vi "chr63204A_Error_conversion.vi"(8 "error in (no error)":errorcluster, 11 "VISA resource name":refnum<visa-resource-name>) -> (0 "error out":errorcluster, 3 "VISA resource name out":refnum<visa-resource-name>)   [LabVIEW 2020]
doc: "This VI converts chr63204A machine errors to LabView errors"
panel:
  out "PROT?":bool[](array[boolean])
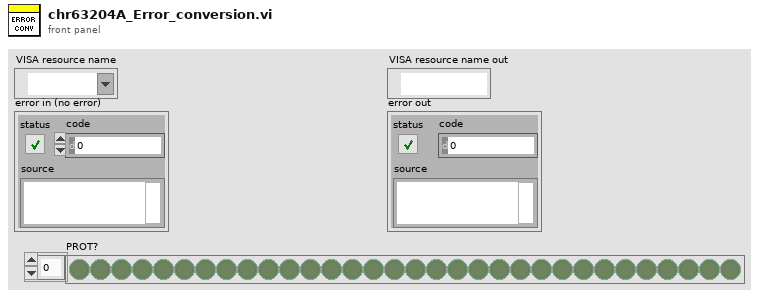
[diagram p1: front panel]
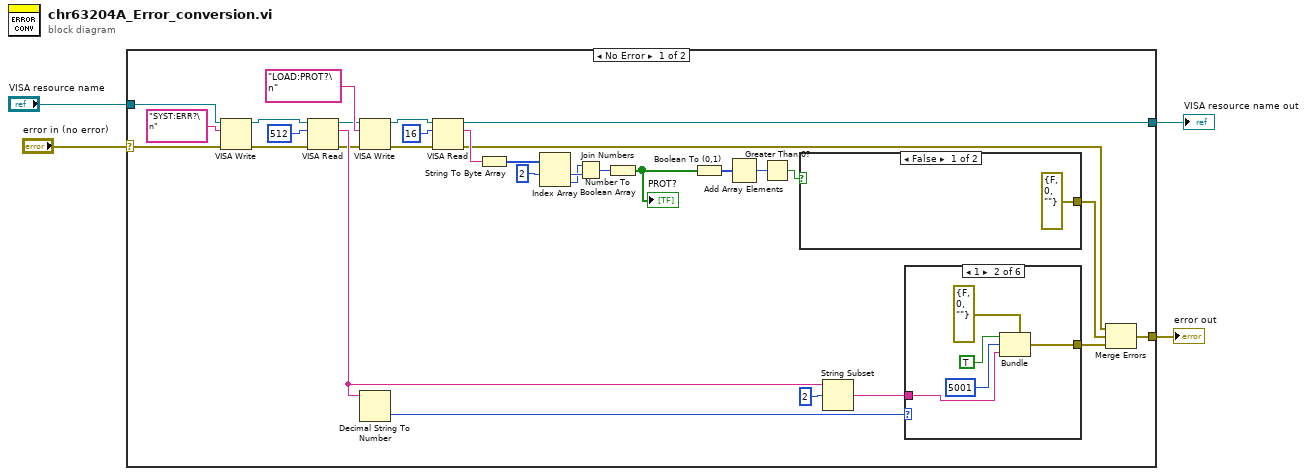
[diagram p0: block diagram]
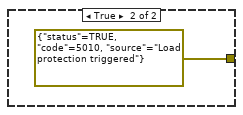
[diagram p2: hidden frame]
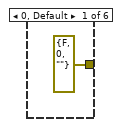
[diagram p3: hidden frame]
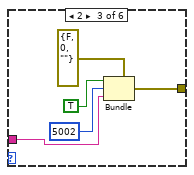
[diagram p4: hidden frame]
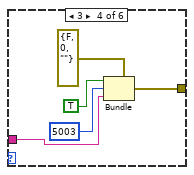
[diagram p5: hidden frame]
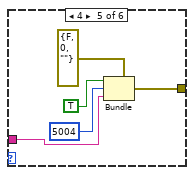
[diagram p6: hidden frame]
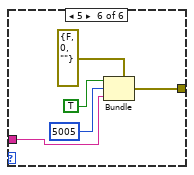
[diagram p7: hidden frame]
diagram:
  n1 = case shown="No Error" "error in (no error)" {
    selector: "error in (no error)" -> [w26 w64]
    tunnel: "VISA resource name" -> [w30 w65]
    tunnel: [w24 w64] -> w1
    tunnel: [w8 w65] -> w2
    frame No Error {
      n2 = VISA Write(VISA resource name=w30, write buffer="SYST:ERR?\n" ("Write Buffer"), error in (no error)=w26) -> (VISA resource name out=w29:refnum<visa-resource-name>, error out=w28:errorcluster)  [unwired: 1 out]
      n3 = VISA Read(VISA resource name=w29, byte count=u32 512, error in (no error)=w28) -> (VISA resource name out=w9:refnum<visa-resource-name>, read buffer=w27:string, error out=w10:errorcluster)  [unwired: 1 out]
      n4 = VISA Write(VISA resource name=w9, write buffer="LOAD:PROT?\n", error in (no error)=w10) -> (VISA resource name out=w21:refnum<visa-resource-name>, error out=w20:errorcluster)  [unwired: 1 out]
      n5 = Decimal String To Number(string=w27) -> (number=w35:i32)  [unwired: 2 in, 1 out]
      n6 = VISA Read(VISA resource name=w21, byte count=u32 16, error in (no error)=w20) -> (VISA resource name out=w8:refnum<visa-resource-name>, read buffer=w18:string, error out=w5:errorcluster)  [unwired: 1 out]
      n7 = String To Byte Array(string=w18) -> (unsigned byte array=w23:u8[])
      n8 = Index Array(array=w23, index #1=2 ("y")) -> (element #1=w22:u8, element #2=w16:u8)  [unwired: 1 in]
      n9 = Join Numbers(hi=w16, lo=w22) -> ((hi.lo)=w15:u16)
      n10 = Number To Boolean Array(number=w15) -> (Boolean array=w14:bool[])
      "PROT?" <- w14
      n11 = Boolean To (0,1)(Boolean=w14) -> (0, 1=w13:i16[])
      n12 = Add Array Elements(numeric array=w13) -> (sum=w12:i16)
      n13 = Greater Than 0?(x=w12) -> (x > 0?=w7:bool)
      n14 = case shown="False" w7 {
        tunnel: [errorcluster {"status"=FALSE, "code"=0, "source"=""} ("error constant") errorcluster {"status"=TRUE, "code"=5010, "source"="Load protection triggered"} ("error constant")] -> w6
        frame False {
        }
        frame True {
        }
      }
      n15 = String Subset(string=w27, offset (0)=2) -> (substring=w33:string)  [unwired: 1 in]
      n16 = case shown="1" w35 {
        tunnel: w33 -> [_ w40 w45 w50 w55 w60]
        tunnel: [errorcluster {"status"=FALSE, "code"=0, "source"=""} ("error constant") w39 w44 w49 w54 w59] -> w25
        frame 0, Default {
        }
        frame 1 {
          n17 = Bundle(cluster=errorcluster {"status"=FALSE, "code"=0, "source"=""} ("error constant"), "status"=TRUE, "code"=5001, "source"=w40) -> (w39:errorcluster)
        }
        frame 2 {
          n18 = Bundle(cluster=errorcluster {"status"=FALSE, "code"=0, "source"=""} ("error constant"), "status"=TRUE, "code"=5002, "source"=w45) -> (w44:errorcluster)
        }
        frame 3 {
          n19 = Bundle(cluster=errorcluster {"status"=FALSE, "code"=0, "source"=""} ("error constant"), "status"=TRUE, "code"=5003, "source"=w50) -> (w49:errorcluster)
        }
        frame 4 {
          n20 = Bundle(cluster=errorcluster {"status"=FALSE, "code"=0, "source"=""} ("error constant"), "status"=TRUE, "code"=5004, "source"=w55) -> (w54:errorcluster)
        }
        frame 5 {
          n21 = Bundle(cluster=errorcluster {"status"=FALSE, "code"=0, "source"=""} ("error constant"), "status"=TRUE, "code"=5005, "source"=w60) -> (w59:errorcluster)
        }
      }
      n22 = Merge Errors(w5, w6, w25) -> (w24:errorcluster)
    }
    frame Error {
    }
  }
  "VISA resource name out" <- w2
  "error out" <- w1
